vi "FinalizeTurn.vi"(6 "Error":errorcluster, 7 "BaseActor":refnum<class "BaseActor.lvclass">) -> (4 "Error":errorcluster, 5 "BaseActor":refnum<class "BaseActor.lvclass">)   [LabVIEW 2020, in "jettl.lvlib" / "BaseActor.lvlib" / "BaseActor.lvclass"]
uses:
  BaseActor.lvclass
  BaseActor.lvclass/BaseActor.ctl
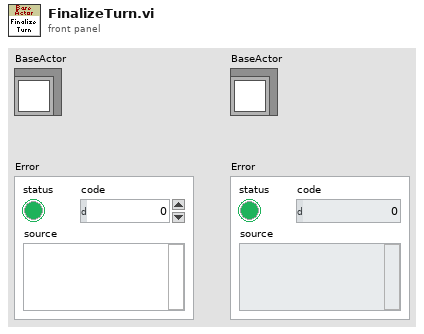
[diagram p1: front panel]
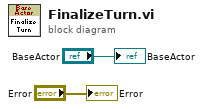
[diagram p0: block diagram]
diagram:
  "BaseActor" <- "BaseActor"
  "Error" <- "Error"
